vi "Lab Panel V5.29.vi"() -> ()   [LabVIEW 2013] (continued)
                n1113 = Unbundle(w2127) -> ("STATUS"=w2121:string)  [unwired: 2 out]
                n1114 = Equal?(x=w2121, y="RUN") -> (x = y?=w2123:bool)
                n1115 = And(x=w2123, y=w2124) -> (x .and. y?=w2122:bool)
                n1116 = case shown="True" w2122 {
                  tunnel: w2127 -> [_ w2132]
                  tunnel: w2126 -> [_ w2136]
                  frame False {
                  }
                  frame True {
                    n1117 = local read "SET LAB01-1"() -> (w2138:T5)
                    n1118 = local read "TDMS LAB01-1"() -> (w2131:refnum<k34>)
                    n1119 = Unbundle(w2138) -> ("CYCLES"=w2129:dbl, "T-RISE mins"=w2135:dbl)  [unwired: 3 out]
                    n1120 = case shown="\"CYCLE TEST\"" w2136 {
                      tunnel: w2135 -> [_ _ w2145]
                      tunnel: [w2140 w2142 w2145] -> w2134
                      tunnel: w2129 -> [w2140 w2142 _]
                      tunnel: ["CHART PASS" "CYCLE PASS" "T-RISE PASS"] -> w2133
                      frame "CHART TEST", Default {
                      }
                      frame "CYCLE TEST" {
                      }
                      frame "T-RISE TEST" {
                      }
                    }
                    n1121 = Unbundle(w2132) -> ("CYCLE"=w2137:dbl)  [unwired: 2 out]
                    n1122 = Increment(x=w2129) -> (x+1=w2130:dbl)
                    n1123 = Greater Or Equal?(x=w2137, y=w2130) -> (x >= y?=w2139:bool)
                    n1124 = case shown="True" w2139 {
                      tunnel: w2134 -> [w2149 _]
                      tunnel: w2133 -> [w2148 _]
                      tunnel: w2132 -> [w2147 _]
                      tunnel: w2131 -> [w2146 _]
                      frame True {
                        n1125 = stacked-sequence {
                          tunnel: w2149 -> [w2153 _]
                          tunnel: w2148 -> [w2151 w2157]
                          tunnel: w2147 -> [_ w2160]
                          tunnel: w2146 -> [w2150 _]
                          frame #0 {
                            n1126 = Build Array(w2151) -> (w2154:string[])
                            n1127 = Build Array(w2153) -> (w2152:dbl[])
                            n1128 = TDMS Write(0:w2150, 5:"TEST PASS", 7:w2154, 9:w2152) -> (15:w2156:errorcluster)  [unwired: 2 in, 3 out]
                            n1129 = local write "data file error"(w2156) -> ()
                          }
                          frame #1 {
                            n1130 = Bundle(cluster=w2160, "STATUS"=w2157) -> (w2158:T4)  [unwired: 2 in]
                            n1131 = local write "RESULT LAB01-1"(TRUE) -> ()
                            n1132 = local write "DISP LAB01-1"(w2158) -> ()
                          }
                        }
                      }
                      frame False {
                      }
                    }
                  }
                }
              }
              frame #1 {
                # "LAB01-2"
                n1133 = Less?(x=w2161, y=2) -> (x < y?=w2164:bool)
                n1134 = local read "DISP LAB01-2"() -> (w2166:T4)
                n1135 = Unbundle(w2166) -> ("STATUS"=w2167:string)  [unwired: 2 out]
                n1136 = Equal?(x=w2167, y="RUN") -> (x = y?=w2163:bool)
                n1137 = And(x=w2163, y=w2164) -> (x .and. y?=w2162:bool)
                n1138 = case shown="True" w2162 {
                  tunnel: w2166 -> [_ w2172]
                  tunnel: w2161 -> [_ w2176]
                  frame False {
                  }
                  frame True {
                    n1139 = local read "SET LAB01-2"() -> (w2178:T5)
                    n1140 = local read "TDMS LAB01-2"() -> (w2171:refnum<k34>)
                    n1141 = Unbundle(w2178) -> ("CYCLES"=w2169:dbl, "T-RISE mins"=w2175:dbl)  [unwired: 3 out]
                    n1142 = case shown="\"T-RISE TEST\"" w2176 {
                      tunnel: w2175 -> [_ _ w2185]
                      tunnel: [w2180 w2182 w2185] -> w2174
                      tunnel: w2169 -> [w2180 w2182 _]
                      tunnel: ["CHART PASS" "CYCLE PASS" "T-RISE PASS"] -> w2173
                      frame "CHART TEST", Default {
                      }
                      frame "CYCLE TEST" {
                      }
                      frame "T-RISE TEST" {
                      }
                    }
                    n1143 = Unbundle(w2172) -> ("CYCLE"=w2177:dbl)  [unwired: 2 out]
                    n1144 = Increment(x=w2169) -> (x+1=w2170:dbl)
                    n1145 = Greater Or Equal?(x=w2177, y=w2170) -> (x >= y?=w2179:bool)
                    n1146 = case shown="True" w2179 {
                      tunnel: w2174 -> [w2189 _]
                      tunnel: w2173 -> [w2188 _]
                      tunnel: w2172 -> [w2187 _]
                      tunnel: w2171 -> [w2186 _]
                      frame True {
                        n1147 = stacked-sequence {
                          tunnel: w2189 -> [w2193 _]
                          tunnel: w2188 -> [w2191 w2197]
                          tunnel: w2187 -> [_ w2200]
                          tunnel: w2186 -> [w2190 _]
                          frame #0 {
                            n1148 = Build Array(w2191) -> (w2194:string[])
                            n1149 = Build Array(w2193) -> (w2192:dbl[])
                            n1150 = TDMS Write(0:w2190, 5:"TEST PASS", 7:w2194, 9:w2192) -> (15:w2196:errorcluster)  [unwired: 2 in, 3 out]
                            n1151 = local write "data file error"(w2196) -> ()
                          }
                          frame #1 {
                            n1152 = Bundle(cluster=w2200, "STATUS"=w2197) -> (w2198:T4)  [unwired: 2 in]
                            n1153 = local write "RESULT LAB01-2"(TRUE) -> ()
                            n1154 = local write "DISP LAB01-2"(w2198) -> ()
                          }
                        }
                      }
                      frame False {
                      }
                    }
                  }
                }
              }
              frame #2 {
                # "LAB02-1"
                n1155 = Less?(x=w2201, y=2) -> (x < y?=w2204:bool)
                n1156 = local read "DISP LAB02-1"() -> (w2206:T4)
                n1157 = Unbundle(w2206) -> ("STATUS"=w2207:string)  [unwired: 2 out]
                n1158 = Equal?(x=w2207, y="RUN") -> (x = y?=w2203:bool)
                n1159 = And(x=w2203, y=w2204) -> (x .and. y?=w2202:bool)
                n1160 = case shown="True" w2202 {
                  tunnel: w2206 -> [_ w2212]
                  tunnel: w2201 -> [_ w2216]
                  frame False {
                  }
                  frame True {
                    n1161 = local read "SET LAB02-1"() -> (w2218:T5)
                    n1162 = local read "TDMS LAB02-1"() -> (w2211:refnum<k34>)
                    n1163 = Unbundle(w2212) -> ("CYCLE"=w2217:dbl)  [unwired: 2 out]
                    n1164 = Unbundle(w2218) -> ("CYCLES"=w2209:dbl, "T-RISE mins"=w2215:dbl)  [unwired: 3 out]
                    n1165 = case shown="\"T-RISE TEST\"" w2216 {
                      tunnel: w2215 -> [_ _ w2225]
                      tunnel: [w2220 w2222 w2225] -> w2214
                      tunnel: w2209 -> [w2220 w2222 _]
                      tunnel: ["CHART PASS" "CYCLE PASS" "T-RISE PASS"] -> w2213
                      frame "CHART TEST", Default {
                      }
                      frame "CYCLE TEST" {
                      }
                      frame "T-RISE TEST" {
                      }
                    }
                    n1166 = Increment(x=w2209) -> (x+1=w2210:dbl)
                    n1167 = Greater Or Equal?(x=w2217, y=w2210) -> (x >= y?=w2219:bool)
                    n1168 = case shown="True" w2219 {
                      tunnel: w2214 -> [w2229 _]
                      tunnel: w2213 -> [w2228 _]
                      tunnel: w2212 -> [w2227 _]
                      tunnel: w2211 -> [w2226 _]
                      frame True {
                        n1169 = stacked-sequence {
                          tunnel: w2229 -> [w2233 _]
                          tunnel: w2228 -> [w2231 w2237]
                          tunnel: w2227 -> [_ w2240]
                          tunnel: w2226 -> [w2230 _]
                          frame #0 {
                            n1170 = Build Array(w2231) -> (w2234:string[])
                            n1171 = Build Array(w2233) -> (w2232:dbl[])
                            n1172 = TDMS Write(0:w2230, 5:"TEST PASS", 7:w2234, 9:w2232) -> (15:w2236:errorcluster)  [unwired: 2 in, 3 out]
                            n1173 = local write "data file error"(w2236) -> ()
                          }
                          frame #1 {
                            n1174 = Bundle(cluster=w2240, "STATUS"=w2237) -> (w2238:T4)  [unwired: 2 in]
                            n1175 = local write "RESULT LAB02-1"(TRUE) -> ()
                            n1176 = local write "DISP LAB02-1"(w2238) -> ()
                          }
                        }
                      }
                      frame False {
                      }
                    }
                  }
                }
              }
              frame #3 {
                # "LAB02-2"
                n1177 = Less?(x=w2241, y=2) -> (x < y?=w2244:bool)
                n1178 = local read "DISP LAB02-2"() -> (w2246:T4)
                n1179 = Unbundle(w2246) -> ("STATUS"=w2247:string)  [unwired: 2 out]
                n1180 = Equal?(x=w2247, y="RUN") -> (x = y?=w2243:bool)
                n1181 = And(x=w2243, y=w2244) -> (x .and. y?=w2242:bool)
                n1182 = case shown="True" w2242 {
                  tunnel: w2246 -> [_ w2252]
                  tunnel: w2241 -> [_ w2256]
                  frame False {
                  }
                  frame True {
                    n1183 = local read "SET LAB02-2"() -> (w2258:T5)
                    n1184 = local read "TDMS LAB02-2"() -> (w2251:refnum<k34>)
                    n1185 = Unbundle(w2252) -> ("CYCLE"=w2257:dbl)  [unwired: 2 out]
                    n1186 = Unbundle(w2258) -> ("CYCLES"=w2249:dbl, "T-RISE mins"=w2255:dbl)  [unwired: 3 out]
                    n1187 = case shown="\"T-RISE TEST\"" w2256 {
                      tunnel: w2255 -> [_ _ w2265]
                      tunnel: [w2260 w2262 w2265] -> w2254
                      tunnel: w2249 -> [w2260 w2262 _]
                      tunnel: ["CHART PASS" "CYCLE PASS" "T-RISE PASS"] -> w2253
                      frame "CHART TEST", Default {
                      }
                      frame "CYCLE TEST" {
                      }
                      frame "T-RISE TEST" {
                      }
                    }
                    n1188 = Increment(x=w2249) -> (x+1=w2250:dbl)
                    n1189 = Greater Or Equal?(x=w2257, y=w2250) -> (x >= y?=w2259:bool)
                    n1190 = case shown="True" w2259 {
                      tunnel: w2254 -> [w2269 _]
                      tunnel: w2253 -> [w2268 _]
                      tunnel: w2252 -> [w2267 _]
                      tunnel: w2251 -> [w2266 _]
                      frame True {
                        n1191 = stacked-sequence {
                          tunnel: w2269 -> [w2273 _]
                          tunnel: w2268 -> [w2271 w2277]
                          tunnel: w2267 -> [_ w2280]
                          tunnel: w2266 -> [w2270 _]
                          frame #0 {
                            n1192 = Build Array(w2271) -> (w2274:string[])
                            n1193 = Build Array(w2273) -> (w2272:dbl[])
                            n1194 = TDMS Write(0:w2270, 5:"TEST PASS", 7:w2274, 9:w2272) -> (15:w2276:errorcluster)  [unwired: 2 in, 3 out]
                            n1195 = local write "data file error"(w2276) -> ()
                          }
                          frame #1 {
                            n1196 = Bundle(cluster=w2280, "STATUS"=w2277) -> (w2278:T4)  [unwired: 2 in]
                            n1197 = local write "RESULT LAB02-2"(TRUE) -> ()
                            n1198 = local write "DISP LAB02-2"(w2278) -> ()
                          }
                        }
                      }
                      frame False {
                      }
                    }
                  }
                }
              }
              frame #4 {
                # "LAB03-1"
                n1199 = Less?(x=w2281, y=2) -> (x < y?=w2284:bool)
                n1200 = local read "DISP LAB03-1"() -> (w2286:T4)
                n1201 = Unbundle(w2286) -> ("STATUS"=w2287:string)  [unwired: 2 out]
                n1202 = Equal?(x=w2287, y="RUN") -> (x = y?=w2283:bool)
                n1203 = And(x=w2283, y=w2284) -> (x .and. y?=w2282:bool)
                n1204 = case shown="True" w2282 {
                  tunnel: w2286 -> [_ w2292]
                  tunnel: w2281 -> [_ w2296]
                  frame False {
                  }
                  frame True {
                    n1205 = local read "SET LAB03-1"() -> (w2298:T5)
                    n1206 = local read "TDMS LAB03-1"() -> (w2291:refnum<k34>)
                    n1207 = Unbundle(w2292) -> ("CYCLE"=w2297:dbl)  [unwired: 2 out]
                    n1208 = Unbundle(w2298) -> ("CYCLES"=w2289:dbl, "T-RISE mins"=w2295:dbl)  [unwired: 3 out]
                    n1209 = case shown="\"T-RISE TEST\"" w2296 {
                      tunnel: w2295 -> [_ _ w2305]
                      tunnel: [w2300 w2302 w2305] -> w2294
                      tunnel: w2289 -> [w2300 w2302 _]
                      tunnel: ["CHART PASS" "CYCLE PASS" "T-RISE PASS"] -> w2293
                      frame "CHART TEST", Default {
                      }
                      frame "CYCLE TEST" {
                      }
                      frame "T-RISE TEST" {
                      }
                    }
                    n1210 = Increment(x=w2289) -> (x+1=w2290:dbl)
                    n1211 = Greater Or Equal?(x=w2297, y=w2290) -> (x >= y?=w2299:bool)
                    n1212 = case shown="True" w2299 {
                      tunnel: w2294 -> [w2309 _]
                      tunnel: w2293 -> [w2308 _]
                      tunnel: w2292 -> [w2307 _]
                      tunnel: w2291 -> [w2306 _]
                      frame True {
                        n1213 = stacked-sequence {
                          tunnel: w2309 -> [w2313 _]
                          tunnel: w2308 -> [w2311 w2317]
                          tunnel: w2307 -> [_ w2320]
                          tunnel: w2306 -> [w2310 _]
                          frame #0 {
                            n1214 = Build Array(w2311) -> (w2314:string[])
                            n1215 = Build Array(w2313) -> (w2312:dbl[])
                            n1216 = TDMS Write(0:w2310, 5:"TEST PASS", 7:w2314, 9:w2312) -> (15:w2316:errorcluster)  [unwired: 2 in, 3 out]
                            n1217 = local write "data file error"(w2316) -> ()
                          }
                          frame #1 {
                            n1218 = Bundle(cluster=w2320, "STATUS"=w2317) -> (w2318:T4)  [unwired: 2 in]
                            n1219 = local write "RESULT LAB03-1"(TRUE) -> ()
                            n1220 = local write "DISP LAB03-1"(w2318) -> ()
                          }
                        }
                      }
                      frame False {
                      }
                    }
                  }
                }
              }
              frame #5 {
                # "LAB03-2"
                n1221 = Less?(x=w2321, y=2) -> (x < y?=w2324:bool)
                n1222 = local read "DISP LAB03-2"() -> (w2326:T4)
                n1223 = Unbundle(w2326) -> ("STATUS"=w2327:string)  [unwired: 2 out]
                n1224 = Equal?(x=w2327, y="RUN") -> (x = y?=w2323:bool)
                n1225 = And(x=w2323, y=w2324) -> (x .and. y?=w2322:bool)
                n1226 = case shown="True" w2322 {
                  tunnel: w2326 -> [_ w2332]
                  tunnel: w2321 -> [_ w2336]
                  frame False {
                  }
                  frame True {
                    n1227 = local read "SET LAB03-2"() -> (w2338:T5)
                    n1228 = local read "TDMS LAB03-2"() -> (w2331:refnum<k34>)
                    n1229 = Unbundle(w2332) -> ("CYCLE"=w2337:dbl)  [unwired: 2 out]
                    n1230 = Unbundle(w2338) -> ("CYCLES"=w2329:dbl, "T-RISE mins"=w2335:dbl)  [unwired: 3 out]
                    n1231 = case shown="\"T-RISE TEST\"" w2336 {
                      tunnel: w2335 -> [_ _ w2345]
                      tunnel: [w2340 w2342 w2345] -> w2334
                      tunnel: w2329 -> [w2340 w2342 _]
                      tunnel: ["CHART PASS" "CYCLE PASS" "T-RISE PASS"] -> w2333
                      frame "CHART TEST", Default {
                      }
                      frame "CYCLE TEST" {
                      }
                      frame "T-RISE TEST" {
                      }
                    }
                    n1232 = Increment(x=w2329) -> (x+1=w2330:dbl)
                    n1233 = Greater Or Equal?(x=w2337, y=w2330) -> (x >= y?=w2339:bool)
                    n1234 = case shown="True" w2339 {
                      tunnel: w2334 -> [w2349 _]
                      tunnel: w2333 -> [w2348 _]
                      tunnel: w2332 -> [w2347 _]
                      tunnel: w2331 -> [w2346 _]
                      frame True {
                        n1235 = stacked-sequence {
                          tunnel: w2349 -> [w2353 _]
                          tunnel: w2348 -> [w2351 w2357]
                          tunnel: w2347 -> [_ w2360]
                          tunnel: w2346 -> [w2350 _]
                          frame #0 {
                            n1236 = Build Array(w2351) -> (w2354:string[])
                            n1237 = Build Array(w2353) -> (w2352:dbl[])
                            n1238 = TDMS Write(0:w2350, 5:"TEST PASS", 7:w2354, 9:w2352) -> (15:w2356:errorcluster)  [unwired: 2 in, 3 out]
                            n1239 = local write "data file error"(w2356) -> ()
                          }
                          frame #1 {
                            n1240 = Bundle(cluster=w2360, "STATUS"=w2357) -> (w2358:T4)  [unwired: 2 in]
                            n1241 = local write "RESULT LAB03-2"(TRUE) -> ()
                            n1242 = local write "DISP LAB03-2"(w2358) -> ()
                          }
                        }
                      }
                      frame False {
                      }
                    }
                  }
                }
              }
              frame #6 {
                # "LAB04-1"
                n1243 = Less?(x=w2361, y=2) -> (x < y?=w2364:bool)
                n1244 = local read "DISP LAB04-1"() -> (w2366:T4)
                n1245 = Unbundle(w2366) -> ("STATUS"=w2367:string)  [unwired: 2 out]
                n1246 = Equal?(x=w2367, y="RUN") -> (x = y?=w2363:bool)
                n1247 = And(x=w2363, y=w2364) -> (x .and. y?=w2362:bool)
                n1248 = case shown="True" w2362 {
                  tunnel: w2366 -> [_ w2372]
                  tunnel: w2361 -> [_ w2376]
                  frame False {
                  }
                  frame True {
                    n1249 = local read "SET LAB04-1"() -> (w2378:T5)
                    n1250 = local read "TDMS LAB04-1"() -> (w2371:refnum<k34>)
                    n1251 = Unbundle(w2372) -> ("CYCLE"=w2377:dbl)  [unwired: 2 out]
                    n1252 = Unbundle(w2378) -> ("CYCLES"=w2369:dbl, "T-RISE mins"=w2375:dbl)  [unwired: 3 out]
                    n1253 = case shown="\"T-RISE TEST\"" w2376 {
                      tunnel: w2375 -> [_ _ w2385]
                      tunnel: [w2380 w2382 w2385] -> w2374
                      tunnel: w2369 -> [w2380 w2382 _]
                      tunnel: ["CHART PASS" "CYCLE PASS" "T-RISE PASS"] -> w2373
                      frame "CHART TEST", Default {
                      }
                      frame "CYCLE TEST" {
                      }
                      frame "T-RISE TEST" {
                      }
                    }
                    n1254 = Increment(x=w2369) -> (x+1=w2370:dbl)
                    n1255 = Greater Or Equal?(x=w2377, y=w2370) -> (x >= y?=w2379:bool)
                    n1256 = case shown="True" w2379 {
                      tunnel: w2374 -> [w2389 _]
                      tunnel: w2373 -> [w2388 _]
                      tunnel: w2372 -> [w2387 _]
                      tunnel: w2371 -> [w2386 _]
                      frame True {
                        n1257 = stacked-sequence {
                          tunnel: w2389 -> [w2393 _]
                          tunnel: w2388 -> [w2391 w2397]
                          tunnel: w2387 -> [_ w2400]
                          tunnel: w2386 -> [w2390 _]
                          frame #0 {
                            n1258 = Build Array(w2391) -> (w2394:string[])
                            n1259 = Build Array(w2393) -> (w2392:dbl[])
                            n1260 = TDMS Write(0:w2390, 5:"TEST PASS", 7:w2394, 9:w2392) -> (15:w2396:errorcluster)  [unwired: 2 in, 3 out]
                            n1261 = local write "data file error"(w2396) -> ()
                          }
                          frame #1 {
                            n1262 = Bundle(cluster=w2400, "STATUS"=w2397) -> (w2398:T4)  [unwired: 2 in]
                            n1263 = local write "RESULT LAB04-1"(TRUE) -> ()
                            n1264 = local write "DISP LAB04-1"(w2398) -> ()
                          }
                        }
                      }
                      frame False {
                      }
                    }
                  }
                }
              }
              frame #7 {
                # "LAB04-2"
                n1265 = Less?(x=w2401, y=2) -> (x < y?=w2404:bool)
                n1266 = local read "DISP LAB04-2"() -> (w2406:T4)
                n1267 = Unbundle(w2406) -> ("STATUS"=w2407:string)  [unwired: 2 out]
                n1268 = Equal?(x=w2407, y="RUN") -> (x = y?=w2403:bool)
                n1269 = And(x=w2403, y=w2404) -> (x .and. y?=w2402:bool)
                n1270 = case shown="True" w2402 {
                  tunnel: w2406 -> [_ w2412]
                  tunnel: w2401 -> [_ w2416]
                  frame False {
                  }
                  frame True {
                    n1271 = local read "SET LAB04-2"() -> (w2418:T5)
                    n1272 = local read "TDMS LAB04-2"() -> (w2411:refnum<k34>)
                    n1273 = Unbundle(w2412) -> ("CYCLE"=w2417:dbl)  [unwired: 2 out]
                    n1274 = Unbundle(w2418) -> ("CYCLES"=w2409:dbl, "T-RISE mins"=w2415:dbl)  [unwired: 3 out]
                    n1275 = case shown="\"T-RISE TEST\"" w2416 {
                      tunnel: w2415 -> [_ _ w2425]
                      tunnel: [w2420 w2422 w2425] -> w2414
                      tunnel: w2409 -> [w2420 w2422 _]
                      tunnel: ["CHART PASS" "CYCLE PASS" "T-RISE PASS"] -> w2413
                      frame "CHART TEST", Default {
                      }
                      frame "CYCLE TEST" {
                      }
                      frame "T-RISE TEST" {
                      }
                    }
                    n1276 = Increment(x=w2409) -> (x+1=w2410:dbl)
                    n1277 = Greater Or Equal?(x=w2417, y=w2410) -> (x >= y?=w2419:bool)
                    n1278 = case shown="True" w2419 {
                      tunnel: w2414 -> [w2429 _]
                      tunnel: w2413 -> [w2428 _]
                      tunnel: w2412 -> [w2427 _]
                      tunnel: w2411 -> [w2426 _]
                      frame True {
                        n1279 = stacked-sequence {
                          tunnel: w2429 -> [w2433 _]
                          tunnel: w2428 -> [w2431 w2437]
                          tunnel: w2427 -> [_ w2440]
                          tunnel: w2426 -> [w2430 _]
                          frame #0 {
                            n1280 = Build Array(w2431) -> (w2434:string[])
                            n1281 = Build Array(w2433) -> (w2432:dbl[])
                            n1282 = TDMS Write(0:w2430, 5:"TEST PASS", 7:w2434, 9:w2432) -> (15:w2436:errorcluster)  [unwired: 2 in, 3 out]
                            n1283 = local write "data file error"(w2436) -> ()
                          }
                          frame #1 {
                            n1284 = Bundle(cluster=w2440, "STATUS"=w2437) -> (w2438:T4)  [unwired: 2 in]
                            n1285 = local write "RESULT LAB04-2"(TRUE) -> ()
                            n1286 = local write "DISP LAB04-2"(w2438) -> ()
                          }
                        }
                      }
                      frame False {
                      }
                    }
                  }
                }
              }
              frame #8 {
                # "LAB05-1"
                n1287 = Less?(x=w2441, y=2) -> (x < y?=w2444:bool)
                n1288 = local read "DISP LAB05-1"() -> (w2446:T4)
                n1289 = Unbundle(w2446) -> ("STATUS"=w2447:string)  [unwired: 2 out]
                n1290 = Equal?(x=w2447, y="RUN") -> (x = y?=w2443:bool)
                n1291 = And(x=w2443, y=w2444) -> (x .and. y?=w2442:bool)
                n1292 = case shown="True" w2442 {
                  tunnel: w2446 -> [_ w2452]
                  tunnel: w2441 -> [_ w2456]
                  frame False {
                  }
                  frame True {
                    n1293 = local read "SET LAB05-1"() -> (w2458:T5)
                    n1294 = local read "TDMS LAB05-1"() -> (w2451:refnum<k34>)
                    n1295 = Unbundle(w2452) -> ("CYCLE"=w2457:dbl)  [unwired: 2 out]
                    n1296 = Unbundle(w2458) -> ("CYCLES"=w2449:dbl, "T-RISE mins"=w2455:dbl)  [unwired: 3 out]
                    n1297 = case shown="\"T-RISE TEST\"" w2456 {
                      tunnel: w2455 -> [_ _ w2465]
                      tunnel: [w2460 w2462 w2465] -> w2454
                      tunnel: w2449 -> [w2460 w2462 _]
                      tunnel: ["CHART PASS" "CYCLE PASS" "T-RISE PASS"] -> w2453
                      frame "CHART TEST", Default {
                      }
                      frame "CYCLE TEST" {
                      }
                      frame "T-RISE TEST" {
                      }
                    }
                    n1298 = Increment(x=w2449) -> (x+1=w2450:dbl)
                    n1299 = Greater Or Equal?(x=w2457, y=w2450) -> (x >= y?=w2459:bool)
                    n1300 = case shown="True" w2459 {
                      tunnel: w2454 -> [w2469 _]
                      tunnel: w2453 -> [w2468 _]
                      tunnel: w2452 -> [w2467 _]
                      tunnel: w2451 -> [w2466 _]
                      frame True {
                        n1301 = stacked-sequence {
                          tunnel: w2469 -> [w2473 _]
                          tunnel: w2468 -> [w2471 w2477]
                          tunnel: w2467 -> [_ w2480]
                          tunnel: w2466 -> [w2470 _]
                          frame #0 {
                            n1302 = Build Array(w2471) -> (w2474:string[])
                            n1303 = Build Array(w2473) -> (w2472:dbl[])
                            n1304 = TDMS Write(0:w2470, 5:"TEST PASS", 7:w2474, 9:w2472) -> (15:w2476:errorcluster)  [unwired: 2 in, 3 out]
                            n1305 = local write "data file error"(w2476) -> ()
                          }
                          frame #1 {
                            n1306 = Bundle(cluster=w2480, "STATUS"=w2477) -> (w2478:T4)  [unwired: 2 in]
                            n1307 = local write "RESULT LAB05-1"(TRUE) -> ()
                            n1308 = local write "DISP LAB05-1"(w2478) -> ()
                          }
                        }
                      }
                      frame False {
                      }
                    }
                  }
                }
              }
              frame #9 {
                # "LAB05-2"
                n1309 = Less?(x=w2481, y=2) -> (x < y?=w2484:bool)
                n1310 = local read "DISP LAB05-2"() -> (w2486:T4)
                n1311 = Unbundle(w2486) -> ("STATUS"=w2487:string)  [unwired: 2 out]
                n1312 = Equal?(x=w2487, y="RUN") -> (x = y?=w2483:bool)
                n1313 = And(x=w2483, y=w2484) -> (x .and. y?=w2482:bool)
                n1314 = case shown="True" w2482 {
                  tunnel: w2486 -> [_ w2492]
                  tunnel: w2481 -> [_ w2496]
                  frame False {
                  }
                  frame True {
                    n1315 = local read "SET LAB05-2"() -> (w2498:T5)
                    n1316 = local read "TDMS LAB05-2"() -> (w2491:refnum<k34>)
                    n1317 = Unbundle(w2492) -> ("CYCLE"=w2497:dbl)  [unwired: 2 out]
                    n1318 = Unbundle(w2498) -> ("CYCLES"=w2489:dbl, "T-RISE mins"=w2495:dbl)  [unwired: 3 out]
                    n1319 = case shown="\"T-RISE TEST\"" w2496 {
                      tunnel: w2495 -> [_ _ w2505]
                      tunnel: [w2500 w2502 w2505] -> w2494
                      tunnel: w2489 -> [w2500 w2502 _]
                      tunnel: ["CHART PASS" "CYCLE PASS" "T-RISE PASS"] -> w2493
                      frame "CHART TEST", Default {
                      }
                      frame "CYCLE TEST" {
                      }
                      frame "T-RISE TEST" {
                      }
                    }
                    n1320 = Increment(x=w2489) -> (x+1=w2490:dbl)
                    n1321 = Greater Or Equal?(x=w2497, y=w2490) -> (x >= y?=w2499:bool)
                    n1322 = case shown="True" w2499 {
                      tunnel: w2494 -> [w2509 _]
                      tunnel: w2493 -> [w2508 _]
                      tunnel: w2492 -> [w2507 _]
                      tunnel: w2491 -> [w2506 _]
                      frame True {
                        n1323 = stacked-sequence {
                          tunnel: w2509 -> [w2513 _]
                          tunnel: w2508 -> [w2511 w2517]
                          tunnel: w2507 -> [_ w2520]
                          tunnel: w2506 -> [w2510 _]
                          frame #0 {
                            n1324 = Build Array(w2511) -> (w2514:string[])
                            n1325 = Build Array(w2513) -> (w2512:dbl[])
                            n1326 = TDMS Write(0:w2510, 5:"TEST PASS", 7:w2514, 9:w2512) -> (15:w2516:errorcluster)  [unwired: 2 in, 3 out]
                            n1327 = local write "data file error"(w2516) -> ()
                          }
                          frame #1 {
                            n1328 = Bundle(cluster=w2520, "STATUS"=w2517) -> (w2518:T4)  [unwired: 2 in]
                            n1329 = local write "RESULT LAB05-2"(TRUE) -> ()
                            n1330 = local write "DISP LAB05-2"(w2518) -> ()
                          }
                        }
                      }
                      frame False {
                      }
                    }
                  }
                }
              }
            }
          }
          frame #6 {
            # "check if test cycles reached for temperature rise test"
            n1331 = stacked-sequence {
              tunnel: w2550 -> [_ _ _ _ _ _ _ _ _ _]
              tunnel: w2549 -> [_ _ _ _ _ _ _ _ _ _]
              tunnel: w2548 -> [_ _ _ _ _ _ _ _ _ _]
              tunnel: w2547 -> [_ _ _ _ _ _ _ _ _ _]
              tunnel: w2546 -> [_ _ _ _ _ _ _ _ _ _]
              tunnel: w2545 -> [_ _ _ _ _ _ _ _ _ _]
              tunnel: w2544 -> [_ _ _ _ _ _ _ _ _ _]
              tunnel: w2543 -> [_ _ _ _ _ _ _ _ _ _]
              tunnel: w2542 -> [_ _ _ _ _ _ _ _ _ _]
              tunnel: w2541 -> [_ _ _ _ _ _ _ _ _ _]
              tunnel: w2540 -> [w2556 _ _ _ _ _ _ _ _ _]
              tunnel: w2530 -> [w2551 _ _ _ _ _ _ _ _ _]
              tunnel: w2539 -> [_ w2582 _ _ _ _ _ _ _ _]
              tunnel: w2538 -> [_ _ w2612 _ _ _ _ _ _ _]
              tunnel: w2537 -> [_ _ _ w2642 _ _ _ _ _ _]
              tunnel: w2536 -> [_ _ _ _ w2672 _ _ _ _ _]
              tunnel: w2535 -> [_ _ _ _ _ w2702 _ _ _ _]
              tunnel: w2534 -> [_ _ _ _ _ _ w2732 _ _ _]
              tunnel: w2533 -> [_ _ _ _ _ _ _ w2762 _ _]
              tunnel: w2532 -> [_ _ _ _ _ _ _ _ w2792 _]
              tunnel: w2531 -> [_ _ _ _ _ _ _ _ _ w2822]
              tunnel: w2529 -> [_ w2581 _ _ _ _ _ _ _ _]
              tunnel: w2528 -> [_ _ w2611 _ _ _ _ _ _ _]
              tunnel: w2527 -> [_ _ _ w2641 _ _ _ _ _ _]
              tunnel: w2526 -> [_ _ _ _ w2671 _ _ _ _ _]
              tunnel: w2525 -> [_ _ _ _ _ w2701 _ _ _ _]
              tunnel: w2524 -> [_ _ _ _ _ _ w2731 _ _ _]
              tunnel: w2523 -> [_ _ _ _ _ _ _ w2761 _ _]
              tunnel: w2522 -> [_ _ _ _ _ _ _ _ w2791 _]
              tunnel: w2521 -> [_ _ _ _ _ _ _ _ _ w2821]
              frame #0 {
                # "LAB01-1"
                n1332 = Equal?(x=w2556, y=2) -> (x = y?=w2554:bool)
                n1333 = local read "DISP LAB01-1"() -> (w2557:T4)
                n1334 = Unbundle(w2557) -> ("STATUS"=w2558:string)  [unwired: 2 out]
                n1335 = Equal?(x=w2558, y="RUN") -> (x = y?=w2553:bool)
                n1336 = And(x=w2553, y=w2554) -> (x .and. y?=w2552:bool)
                n1337 = case shown="True" w2552 {
                  tunnel: w2557 -> [_ w2561]
                  tunnel: w2551 -> [_ w2564]
                  frame False {
                  }
                  frame True {
                    n1338 = local read "SET LAB01-1"() -> (w2563:T5)
                    n1339 = local read "TDMS LAB01-1"() -> (w2560:refnum<k34>)
                    n1340 = Unbundle(w2561) -> ("CYCLE"=w2565:dbl)  [unwired: 2 out]
                    n1341 = Unbundle(w2563) -> ("T-RISE mins"=w2562:dbl)  [unwired: 4 out]
                    n1342 = Greater Or Equal?(x=w2565, y=w2564) -> (x >= y?=w2566:bool)
                    n1343 = case shown="True" w2566 {
                      tunnel: w2562 -> [w2569 _]
                      tunnel: w2561 -> [w2568 _]
                      tunnel: w2560 -> [w2567 _]
                      frame True {
                        n1344 = stacked-sequence {
                          tunnel: w2569 -> [w2572 _]
                          tunnel: w2568 -> [_ w2577]
                          tunnel: w2567 -> [w2570 _]
                          frame #0 {
                            n1345 = Build Array("T-RISE") -> (w2574:string[])
                            n1346 = Build Array(w2572) -> (w2573:dbl[])
                            n1347 = TDMS Write(0:w2570, 5:"TEST PASS", 7:w2574, 9:w2573) -> (15:w2576:errorcluster)  [unwired: 2 in, 3 out]
                            n1348 = local write "data file error"(w2576) -> ()
                          }
                          frame #1 {
                            n1349 = Bundle(cluster=w2577, "STATUS"="T-RISE PASS") -> (w2579:T4)  [unwired: 2 in]
                            n1350 = local write "RESULT LAB01-1"(TRUE) -> ()
                            n1351 = local write "DISP LAB01-1"(w2579) -> ()
                          }
                        }
                      }
                      frame False {
                      }
                    }
                  }
                }
              }
              frame #1 {
                # "LAB01-2"
                n1352 = Equal?(x=w2582, y=2) -> (x = y?=w2585:bool)
                n1353 = local read "DISP LAB01-2"() -> (w2587:T4)
                n1354 = Unbundle(w2587) -> ("STATUS"=w2588:string)  [unwired: 2 out]
                n1355 = Equal?(x=w2588, y="RUN") -> (x = y?=w2584:bool)
                n1356 = And(x=w2584, y=w2585) -> (x .and. y?=w2583:bool)
                n1357 = case shown="True" w2583 {
                  tunnel: w2587 -> [_ w2591]
                  tunnel: w2581 -> [_ w2594]
                  frame False {
                  }
                  frame True {
                    n1358 = local read "SET LAB01-2"() -> (w2593:T5)
                    n1359 = local read "TDMS LAB01-2"() -> (w2590:refnum<k34>)
                    n1360 = Unbundle(w2591) -> ("CYCLE"=w2595:dbl)  [unwired: 2 out]
                    n1361 = Unbundle(w2593) -> ("T-RISE mins"=w2592:dbl)  [unwired: 4 out]
                    n1362 = Greater Or Equal?(x=w2595, y=w2594) -> (x >= y?=w2596:bool)
                    n1363 = case shown="True" w2596 {
                      tunnel: w2592 -> [w2599 _]
                      tunnel: w2591 -> [w2598 _]
                      tunnel: w2590 -> [w2597 _]
                      frame True {
                        n1364 = stacked-sequence {
                          tunnel: w2599 -> [w2602 _]
                          tunnel: w2598 -> [_ w2607]
                          tunnel: w2597 -> [w2600 _]
                          frame #0 {
                            n1365 = Build Array("T-RISE") -> (w2604:string[])
                            n1366 = Build Array(w2602) -> (w2603:dbl[])
                            n1367 = TDMS Write(0:w2600, 5:"TEST PASS", 7:w2604, 9:w2603) -> (15:w2606:errorcluster)  [unwired: 2 in, 3 out]
                            n1368 = local write "data file error"(w2606) -> ()
                          }
                          frame #1 {
                            n1369 = Bundle(cluster=w2607, "STATUS"="T-RISE PASS") -> (w2609:T4)  [unwired: 2 in]
                            n1370 = local write "RESULT LAB01-2"(TRUE) -> ()
                            n1371 = local write "DISP LAB01-2"(w2609) -> ()
                          }
                        }
                      }
                      frame False {
                      }
                    }
                  }
                }
              }
              frame #2 {
                # "LAB02-1"
                n1372 = Equal?(x=w2612, y=2) -> (x = y?=w2615:bool)
                n1373 = local read "DISP LAB02-1"() -> (w2617:T4)
                n1374 = Unbundle(w2617) -> ("STATUS"=w2618:string)  [unwired: 2 out]
                n1375 = Equal?(x=w2618, y="RUN") -> (x = y?=w2614:bool)
                n1376 = And(x=w2614, y=w2615) -> (x .and. y?=w2613:bool)
                n1377 = case shown="True" w2613 {
                  tunnel: w2617 -> [_ w2621]
                  tunnel: w2611 -> [_ w2624]
                  frame False {
                  }
                  frame True {
                    n1378 = local read "SET LAB02-1"() -> (w2623:T5)
                    n1379 = local read "TDMS LAB02-1"() -> (w2620:refnum<k34>)
                    n1380 = Unbundle(w2621) -> ("CYCLE"=w2625:dbl)  [unwired: 2 out]
                    n1381 = Unbundle(w2623) -> ("T-RISE mins"=w2622:dbl)  [unwired: 4 out]
                    n1382 = Greater Or Equal?(x=w2625, y=w2624) -> (x >= y?=w2626:bool)
                    n1383 = case shown="True" w2626 {
                      tunnel: w2622 -> [w2629 _]
                      tunnel: w2621 -> [w2628 _]
                      tunnel: w2620 -> [w2627 _]
                      frame True {
                        n1384 = stacked-sequence {
                          tunnel: w2629 -> [w2632 _]
                          tunnel: w2628 -> [_ w2637]
                          tunnel: w2627 -> [w2630 _]
                          frame #0 {
                            n1385 = Build Array("T-RISE") -> (w2634:string[])
                            n1386 = Build Array(w2632) -> (w2633:dbl[])
                            n1387 = TDMS Write(0:w2630, 5:"TEST PASS", 7:w2634, 9:w2633) -> (15:w2636:errorcluster)  [unwired: 2 in, 3 out]
                            n1388 = local write "data file error"(w2636) -> ()
                          }
                          frame #1 {
                            n1389 = Bundle(cluster=w2637, "STATUS"="T-RISE PASS") -> (w2639:T4)  [unwired: 2 in]
                            n1390 = local write "RESULT LAB02-1"(TRUE) -> ()
                            n1391 = local write "DISP LAB02-1"(w2639) -> ()
                          }
                        }
                      }
                      frame False {
                      }
                    }
                  }
                }
              }
              frame #3 {
                # "LAB02-2"
                n1392 = Equal?(x=w2642, y=2) -> (x = y?=w2645:bool)
                n1393 = local read "DISP LAB02-2"() -> (w2647:T4)
                n1394 = Unbundle(w2647) -> ("STATUS"=w2648:string)  [unwired: 2 out]
                n1395 = Equal?(x=w2648, y="RUN") -> (x = y?=w2644:bool)
                n1396 = And(x=w2644, y=w2645) -> (x .and. y?=w2643:bool)
                n1397 = case shown="True" w2643 {
                  tunnel: w2647 -> [_ w2651]
                  tunnel: w2641 -> [_ w2654]
                  frame False {
                  }
                  frame True {
                    n1398 = local read "SET LAB02-2"() -> (w2653:T5)
                    n1399 = local read "TDMS LAB02-2"() -> (w2650:refnum<k34>)
                    n1400 = Unbundle(w2651) -> ("CYCLE"=w2655:dbl)  [unwired: 2 out]
                    n1401 = Unbundle(w2653) -> ("T-RISE mins"=w2652:dbl)  [unwired: 4 out]
                    n1402 = Greater Or Equal?(x=w2655, y=w2654) -> (x >= y?=w2656:bool)
                    n1403 = case shown="True" w2656 {
                      tunnel: w2652 -> [w2659 _]
                      tunnel: w2651 -> [w2658 _]
                      tunnel: w2650 -> [w2657 _]
                      frame True {
                        n1404 = stacked-sequence {
                          tunnel: w2659 -> [w2662 _]
                          tunnel: w2658 -> [_ w2667]
                          tunnel: w2657 -> [w2660 _]
                          frame #0 {
                            n1405 = Build Array("T-RISE") -> (w2664:string[])
                            n1406 = Build Array(w2662) -> (w2663:dbl[])
                            n1407 = TDMS Write(0:w2660, 5:"TEST PASS", 7:w2664, 9:w2663) -> (15:w2666:errorcluster)  [unwired: 2 in, 3 out]
                            n1408 = local write "data file error"(w2666) -> ()
                          }
                          frame #1 {
                            n1409 = Bundle(cluster=w2667, "STATUS"="T-RISE PASS") -> (w2669:T4)  [unwired: 2 in]
                            n1410 = local write "RESULT LAB02-2"(TRUE) -> ()
                            n1411 = local write "DISP LAB02-2"(w2669) -> ()
                          }
                        }
                      }
                      frame False {
                      }
                    }
                  }
                }
              }
              frame #4 {
                # "LAB03-1"
                n1412 = Equal?(x=w2672, y=2) -> (x = y?=w2675:bool)
                n1413 = local read "DISP LAB03-1"() -> (w2677:T4)
                n1414 = Unbundle(w2677) -> ("STATUS"=w2678:string)  [unwired: 2 out]
                n1415 = Equal?(x=w2678, y="RUN") -> (x = y?=w2674:bool)
                n1416 = And(x=w2674, y=w2675) -> (x .and. y?=w2673:bool)
                n1417 = case shown="True" w2673 {
                  tunnel: w2677 -> [_ w2681]
                  tunnel: w2671 -> [_ w2684]
                  frame False {
                  }
                  frame True {
                    n1418 = local read "SET LAB03-1"() -> (w2683:T5)
                    n1419 = local read "TDMS LAB03-1"() -> (w2680:refnum<k34>)
                    n1420 = Unbundle(w2681) -> ("CYCLE"=w2685:dbl)  [unwired: 2 out]
                    n1421 = Unbundle(w2683) -> ("T-RISE mins"=w2682:dbl)  [unwired: 4 out]
                    n1422 = Greater Or Equal?(x=w2685, y=w2684) -> (x >= y?=w2686:bool)
                    n1423 = case shown="True" w2686 {
                      tunnel: w2682 -> [w2689 _]
                      tunnel: w2681 -> [w2688 _]
                      tunnel: w2680 -> [w2687 _]
                      frame True {
                        n1424 = stacked-sequence {
                          tunnel: w2689 -> [w2692 _]
                          tunnel: w2688 -> [_ w2697]
                          tunnel: w2687 -> [w2690 _]
                          frame #0 {
                            n1425 = Build Array("T-RISE") -> (w2694:string[])
                            n1426 = Build Array(w2692) -> (w2693:dbl[])
                            n1427 = TDMS Write(0:w2690, 5:"TEST PASS", 7:w2694, 9:w2693) -> (15:w2696:errorcluster)  [unwired: 2 in, 3 out]
                            n1428 = local write "data file error"(w2696) -> ()
                          }
                          frame #1 {
                            n1429 = Bundle(cluster=w2697, "STATUS"="T-RISE PASS") -> (w2699:T4)  [unwired: 2 in]
                            n1430 = local write "RESULT LAB03-1"(TRUE) -> ()
                            n1431 = local write "DISP LAB03-1"(w2699) -> ()
                          }
                        }
                      }
                      frame False {
                      }
                    }
                  }
                }
              }
              frame #5 {
                # "LAB03-2"
                n1432 = Equal?(x=w2702, y=2) -> (x = y?=w2705:bool)
                n1433 = local read "DISP LAB03-2"() -> (w2707:T4)
                n1434 = Unbundle(w2707) -> ("STATUS"=w2708:string)  [unwired: 2 out]
                n1435 = Equal?(x=w2708, y="RUN") -> (x = y?=w2704:bool)
                n1436 = And(x=w2704, y=w2705) -> (x .and. y?=w2703:bool)
                n1437 = case shown="True" w2703 {
                  tunnel: w2707 -> [_ w2711]
                  tunnel: w2701 -> [_ w2714]
                  frame False {
                  }
                  frame True {
                    n1438 = local read "SET LAB03-2"() -> (w2713:T5)
                    n1439 = local read "TDMS LAB03-2"() -> (w2710:refnum<k34>)
                    n1440 = Unbundle(w2711) -> ("CYCLE"=w2715:dbl)  [unwired: 2 out]
                    n1441 = Unbundle(w2713) -> ("T-RISE mins"=w2712:dbl)  [unwired: 4 out]
                    n1442 = Greater Or Equal?(x=w2715, y=w2714) -> (x >= y?=w2716:bool)
                    n1443 = case shown="True" w2716 {
                      tunnel: w2712 -> [w2719 _]
                      tunnel: w2711 -> [w2718 _]
                      tunnel: w2710 -> [w2717 _]
                      frame True {
                        n1444 = stacked-sequence {
                          tunnel: w2719 -> [w2722 _]
                          tunnel: w2718 -> [_ w2727]
                          tunnel: w2717 -> [w2720 _]
                          frame #0 {
                            n1445 = Build Array("T-RISE") -> (w2724:string[])
                            n1446 = Build Array(w2722) -> (w2723:dbl[])
                            n1447 = TDMS Write(0:w2720, 5:"TEST PASS", 7:w2724, 9:w2723) -> (15:w2726:errorcluster)  [unwired: 2 in, 3 out]
                            n1448 = local write "data file error"(w2726) -> ()
                          }
                          frame #1 {
                            n1449 = Bundle(cluster=w2727, "STATUS"="T-RISE PASS") -> (w2729:T4)  [unwired: 2 in]
                            n1450 = local write "RESULT LAB03-2"(TRUE) -> ()
                            n1451 = local write "DISP LAB03-2"(w2729) -> ()
                          }
                        }
                      }
                      frame False {
                      }
                    }
                  }
                }
              }
              frame #6 {
                # "LAB04-1"
                n1452 = Equal?(x=w2732, y=2) -> (x = y?=w2735:bool)
                n1453 = local read "DISP LAB04-1"() -> (w2737:T4)
                n1454 = Unbundle(w2737) -> ("STATUS"=w2738:string)  [unwired: 2 out]
                n1455 = Equal?(x=w2738, y="RUN") -> (x = y?=w2734:bool)
                n1456 = And(x=w2734, y=w2735) -> (x .and. y?=w2733:bool)
                n1457 = case shown="True" w2733 {
                  tunnel: w2737 -> [_ w2741]
                  tunnel: w2731 -> [_ w2744]
                  frame False {
                  }
                  frame True {
                    n1458 = local read "SET LAB04-1"() -> (w2743:T5)
                    n1459 = local read "TDMS LAB04-1"() -> (w2740:refnum<k34>)
                    n1460 = Unbundle(w2741) -> ("CYCLE"=w2745:dbl)  [unwired: 2 out]
                    n1461 = Unbundle(w2743) -> ("T-RISE mins"=w2742:dbl)  [unwired: 4 out]
                    n1462 = Greater Or Equal?(x=w2745, y=w2744) -> (x >= y?=w2746:bool)
                    n1463 = case shown="True" w2746 {
                      tunnel: w2742 -> [w2749 _]
                      tunnel: w2741 -> [w2748 _]
                      tunnel: w2740 -> [w2747 _]
                      frame True {
                        n1464 = stacked-sequence {
                          tunnel: w2749 -> [w2752 _]
                          tunnel: w2748 -> [_ w2757]
                          tunnel: w2747 -> [w2750 _]
                          frame #0 {
                            n1465 = Build Array("T-RISE") -> (w2754:string[])
                            n1466 = Build Array(w2752) -> (w2753:dbl[])
                            n1467 = TDMS Write(0:w2750, 5:"TEST PASS", 7:w2754, 9:w2753) -> (15:w2756:errorcluster)  [unwired: 2 in, 3 out]
